vi "LS330_Init.vi"(8 "error in":errorcluster, 11 "VISA resource name":refnum<visa-resource-name>) -> (0 "error out":errorcluster, 3 "VISA resource name out":refnum<visa-resource-name>)   [LabVIEW 2021]
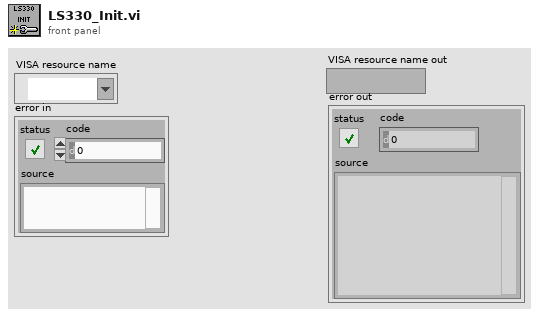
[diagram p1: front panel]
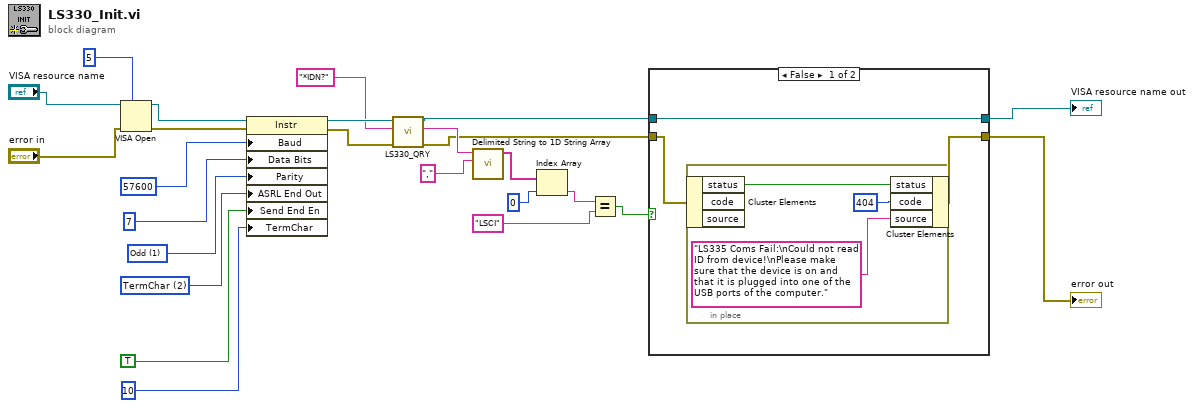
[diagram p0: block diagram]
diagram:
  w17 = u16 2 items=["None", "Last Bit", "TermChar", "Break"] ("Serial Settings:End Mode for Writes")
  w18 = u16 1 items=["None", "Odd", "Even", "Mark", "Space"] ("Serial Settings:Parity")
  n1 = VISA Open(timeout (0)=u32 5 ("VISA Open timeout (0)"), error in (no error)="error in", VISA resource name="VISA resource name") -> (VISA resource name=w22:refnum<visa-resource-name>, error out=w21:errorcluster)  [unwired: 2 in]
  n2 = property class="Instr"(reference=w22, error in=w21, "Baud"=u32 57600 ("Serial Settings:Baud Rate"), "Data Bits"=u16 7 ("Serial Settings:Data Bits"), "Parity"=w18, "ASRL End Out"=w17, "Send End En"=TRUE ("Message Based Settings:Send End Enable"), "TermChar"=u8 10 ("Message Based Settings:Termination Character")) -> (reference out=w14:refnum<visa-resource-name>, error out=w13:errorcluster)
  n3 = call "LS330_QRY.vi"("error in"=w13, "CMD"="*IDN?", "VISA resource name"=w14) -> ("error out"=w4:errorcluster, "OUT"=w11:string, "VISA resource name out"=w3:refnum<visa-resource-name>)  [unwired: 5 in, 1 out]
  n4 = call <vilib>:"Delimited String to 1D String Array.vi"("delimiter"=",", "delimited string"=w11) -> ("string array"=w9:string[])  [unwired: 9 in]
  n5 = Index Array(array=w9, index=0) -> (element=w7:string)
  n6 = Equal?(x=w7, y="LSCI") -> (x = y?=w5:bool)
  n7 = case shown="False" w5 {
    tunnel: w4 -> [w27 w32]
    tunnel: [w28 w33] -> w2
    tunnel: w3 -> [w28 w33]
    tunnel: [w26 w32] -> w1
    frame False {
      n8 = in-place {
        n9 = in-place-cluster #1(w27) -> ("status"=w31:bool)  [unwired: 2 out]
        n10 = in-place-cluster #1("status"=w31, "code"=404, "source"="LS335 Coms Fail:\nCould not read ID from device!\nPlease make sure that the device is on and that it is plugged into one of the USB ports of the computer.") -> (w26:errorcluster)
      }
    }
    frame True {
    }
  }
  "VISA resource name out" <- w2
  "error out" <- w1
